vi "AlgoritmoIntelliplant.vi"() -> ()   [LabVIEW 2020]
uses:
  <vilib>/Analysis/baseanly.llb/Mean (DBL).vi
  <vilib>/Analysis/NI_AALPro.lvlib
  <vilib>/Analysis/NI_AALBase.lvlib
panel:
  out "Economia 2":dbl caption="Numeric 3"
  out "Economia":dbl caption="Numeric 3"
  out "Volume IntelliPlant":dbl
  out "Volume Comum":dbl
  out "Irrigação Intelliplant":dbl(slide) scale=0.0..25.0
  out "Irrigação Comum":dbl(slide) scale=0.0..25.0
  in  "Pluviosidade (mm)":dbl[](array[numeric])=[0.0, 0.0, 0.0, 1.7, 0.3, 0.3]
  in  "Higrometro (%)":dbl[](array[numeric])=[78.0, 73.0, 61.0, 58.0, 56.0, 55.0]
  out "Análise e Previsão de Umidade":cluster{"y vector":dbl[], "y vector":dbl[]}[](graph)
  # "Volume de Água de Irrigação (10³ L/hectare)"
  # "Economia Diária de Água\n                  (10³ L/hectare)"
  # "Economia Mensal de Água\n                  (10³ L/hectare)"
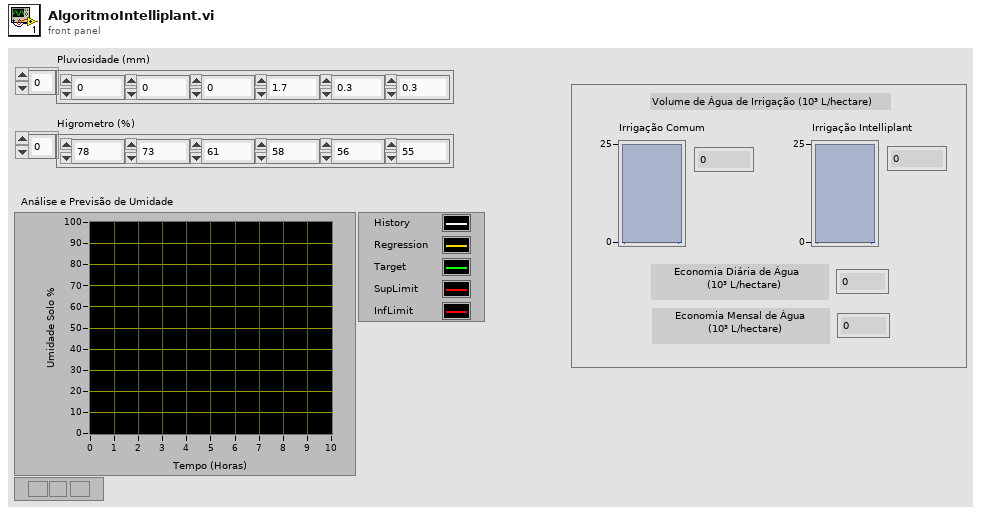
[diagram p1: front panel]
types:
  T1 = cluster{"y vector":dbl[], "Higrometro (%)":dbl[]}
  T2 = cluster{"y vector":dbl[], "Higrometro (%)":dbl[]}[]
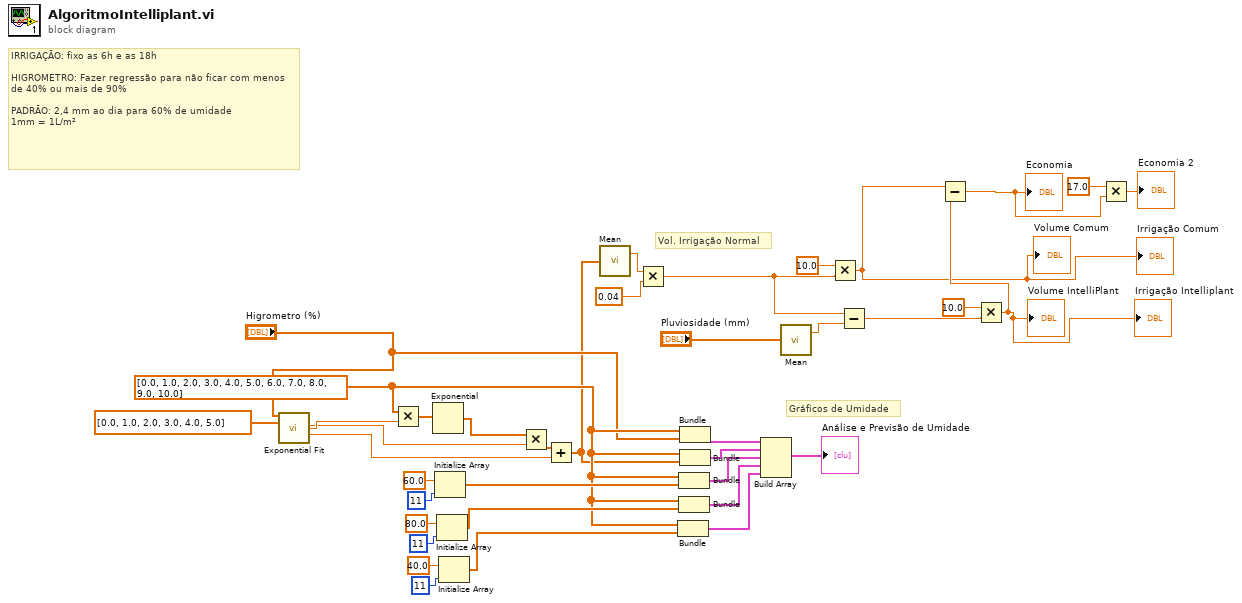
[diagram p0: block diagram]
diagram:
  w23 = dbl[] [0.0, 1.0, 2.0, 3.0, 4.0, 5.0, 6.0, 7.0, 8.0, 9.0, 10.0] ("y vector")
  # "Gráficos de Umidade"
  # "Vol. Irrigação Normal"
  # "IRRIGAÇÃO: fixo as 6h e as 18h\n\nHIGROMETRO: Fazer regressão para não ficar com menos de 40% ou mais de 90%\n\nPADRÃO: 2,4 mm ao dia para 60% de umidade \n1mm = 1L/m²"
  n1 = call <vilib>:"Exponential Fit.vi"("Y"="Higrometro (%)", "X"=dbl[] [0.0, 1.0, 2.0, 3.0, 4.0, 5.0]) -> ("amplitude"=w18:dbl, "damping"=w21:dbl, "offset"=w19:dbl)  [unwired: 8 in, 3 out]
  n2 = Multiply(x=w23, y=w21) -> (x*y=w22:dbl[])
  n3 = Exponential(1:w22) -> (0:w17:dbl[])
  n4 = Initialize Array(60.0 ("element"), 11 ("dimension size")) -> (w26:dbl[])
  n5 = Initialize Array(80.0 ("element"), 11 ("dimension size")) -> (w31:dbl[])
  n6 = Initialize Array(40.0 ("element"), 11 ("dimension size")) -> (w25:dbl[])
  n7 = Multiply(x=w17, y=w18) -> (x*y=w20:dbl[])
  n8 = Add(x=w20, y=w19) -> (x+y=w14:dbl[])
  n9 = call-poly <vilib>:"Mean.vi"("X"=w14) -> ("mean"=w13:dbl)  [unwired: 1 out]
  n10 = Multiply(x=w13, y=0.04) -> (x*y=w4:dbl)
  n11 = Bundle("y vector"=w23, w25) -> (w34:cluster{"y vector":dbl[], dbl[]})  [unwired: 1 in]
  n12 = Bundle("y vector"=w23, w26) -> (w36:cluster{"y vector":dbl[], dbl[]})  [unwired: 1 in]
  n13 = Bundle("y vector"=w23, w31) -> (w35:cluster{"y vector":dbl[], dbl[]})  [unwired: 1 in]
  n14 = Bundle("y vector"=w23, "Higrometro (%)"="Higrometro (%)") -> (w37:T1)  [unwired: 1 in]
  n15 = Bundle("y vector"=w23, w14) -> (w24:cluster{"y vector":dbl[], dbl[]})  [unwired: 1 in]
  n16 = Build Array(w37, w24, w36, w35, w34) -> (→"Análise e Previsão de Umidade":T2)
  n17 = call-poly <vilib>:"Mean.vi"("X"="Pluviosidade (mm)") -> ("mean"=w10:dbl)  [unwired: 1 out]
  n18 = Multiply(x=10.0, y=w4) -> (x*y=w5:dbl)
  "Irrigação Comum" <- w5
  "Volume Comum" <- w5
  n19 = Subtract(x=w4, y=w10) -> (x-y=w7:dbl)
  n20 = Multiply(x=10.0, y=w7) -> (x*y=w6:dbl)
  "Irrigação Intelliplant" <- w6
  "Volume IntelliPlant" <- w6
  n21 = Subtract(x=w5, y=w6) -> (x-y=w1:dbl)
  "Economia" <- w1
  n22 = Multiply(x=17.0, y=w1) -> (x*y=→"Economia 2":dbl)
